vi "Check ElapsedTime.vi"(8 "error in":errorcluster, 11 "Switch in":refnum<class "Switch.lvclass">) -> (0 "error out":errorcluster, 1 "LastSwitch":timestamp, 2 "TimeElapsed?":bool, 3 "Switch out":refnum<class "Switch.lvclass">)   [LabVIEW 2019, in "Switch.lvclass"]
doc: "Check to see if the maximum time has elapsed for a particular state. If so, and the value of the maxElapsedTime is > 0, change the state."
uses:
  Switch.lvclass
  Switch.lvclass/Switch.ctl
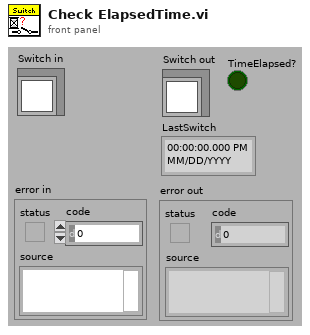
[diagram p1: front panel]
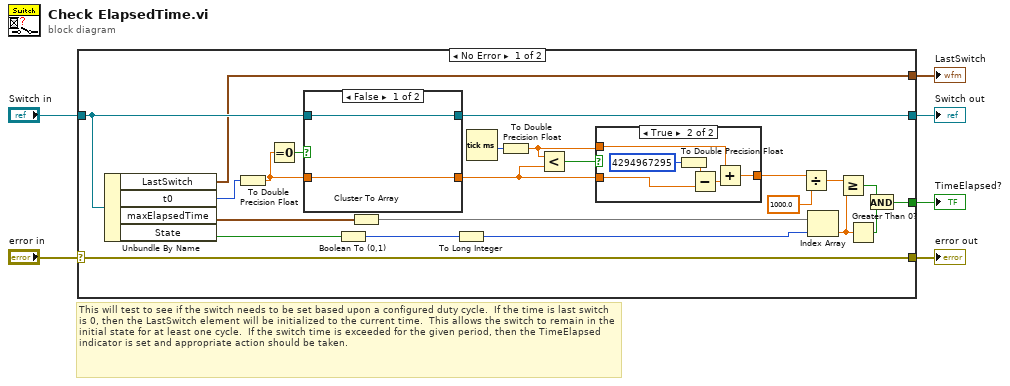
[diagram p0: block diagram]
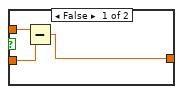
[diagram p2: hidden frame]
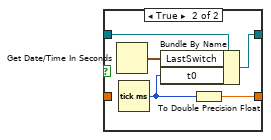
[diagram p3: hidden frame]
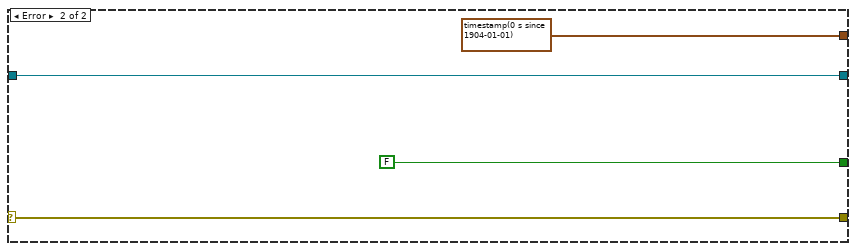
[diagram p4: hidden frame]
diagram:
  # "This will test to see if the switch needs to be set based upon a configured duty cycle.  If the time is last switch is 0, then the LastSwitch element will be initialized to the current time.  This allows the switch to remain in the initial state for at least one cycle.  If the switch time is exceeded for the given period, then the TimeElapsed indicator is set and appropriate action should be taken."
  n1 = case shown="No Error" "error in" {
    selector: "error in" -> [w25 w49]
    tunnel: [w25 w49] -> w5
    tunnel: [w19 w48] -> w3
    tunnel: "Switch in" -> [w20 w48]
    tunnel: [w18 FALSE] -> w1
    tunnel: [w16 timestamp(0 s since 1904-01-01) ("LastSwitch")] -> w2
    frame No Error {
      n2 = Unbundle By Name(w20) -> ("LastSwitch"=w16:timestamp, "t0"=w11:u32, "maxElapsedTime"=w29:cluster{"true":sgl, "false":sgl}, "State"=w17:bool)
      n3 = To Double Precision Float(number=w11) -> (double precision float=w21:dbl)
      n4 = Equal To 0?(x=w21) -> (x = 0?=w22:bool)
      n5 = case shown="False" w22 {
        tunnel: w21 -> [w40 _]
        tunnel: w20 -> [w39 w45]
        tunnel: [w40 w42] -> w8
        tunnel: [w39 w44] -> w19
        frame False {
        }
        frame True {
          n6 = Get Date/Time In Seconds() -> (seconds since 1Jan1904=w43:timestamp)
          n7 = Tick Count (ms)() -> (millisecond timer value=w41:u32)
          n8 = Bundle By Name(cluster=w45, "LastSwitch"=w43, "t0"=w41) -> (w44:refnum<class "Switch.lvclass">)
          n9 = To Double Precision Float(number=w41) -> (double precision float=w42:dbl)
        }
      }
      n10 = Boolean To (0,1)(Boolean=w17) -> (0, 1=w27:i16)
      n11 = Cluster To Array(cluster=w29) -> (array=w28:sgl[])
      n12 = To Long Integer(number=w27) -> (32bit integer=w26:i32)
      n13 = Tick Count (ms)() -> (millisecond timer value=w14:u32)
      n14 = To Double Precision Float(number=w14) -> (double precision float=w9:dbl)
      n15 = Less?(x=w9, y=w8) -> (x < y?=w10:bool)
      n16 = case shown="True" w10 {
        tunnel: w9 -> [w32 w33]
        tunnel: w8 -> [w31 w35]
        tunnel: [w30 w36] -> w7
        frame False {
          n17 = Subtract(x=w32, y=w31) -> (x-y=w30:dbl)
        }
        frame True {
          n18 = To Double Precision Float(number=u32 4294967295 ("millisecond timer value")) -> (double precision float=w37:dbl)
          n19 = Subtract(x=w37, y=w35) -> (x-y=w34:dbl)
          n20 = Add(x=w33, y=w34) -> (x+y=w36:dbl)
        }
      }
      n21 = Divide(x=w7, y=1000.0) -> (x/y=w12:dbl)
      n22 = Index Array(array=w28, index=w26) -> (element=w15:sgl)
      n23 = Greater Or Equal?(x=w12, y=w15) -> (x >= y?=w23:bool)
      n24 = Greater Than 0?(x=w15) -> (x > 0?=w24:bool)
      n25 = And(x=w23, y=w24) -> (x .and. y?=w18:bool)
    }
    frame Error {
    }
  }
  "error out" <- w5
  "Switch out" <- w3
  "TimeElapsed?" <- w1
  "LastSwitch" <- w2
